vi "Main UI.vi"(11 "FormulaLV App in":refnum<class "FormulaG App.lvclass">) -> ()   [LabVIEW 2020, in "FormulaG.lvlib" / "FormulaG App.lvclass"]
uses:
  FormulaG App.lvclass
  <vilib>/sklein/WebView2/Webview2 Control/WebView2 Control.xctl
  FormulaLV-Common/Camera.ctl
  FormulaLV-Common/Car Info.ctl
  FormulaG App.lvclass/FormulaG App.ctl
  FormulaLV-Common/UI Options.ctl
  FormulaLV-Common/FormulaG-Common.lvlib
  FormulaG API/FormulaG API.lvclass
panel:
  out "XY Graph":cluster{dbl[], dbl[]}[](graph)
  out "Info":T1 {"Heading" format="%.2f"; "Y" format="%.2f"; "X" format="%.2f"; "Speed" format="%.2f"}
  in  "Pause":bool
  in  "Sensitivity":sgl(slide)=0.5148515 scale=0.0..1.0
  out "Chart":sgl[][](graph)
  in  "Camera":T2
  in  "Reset":bool
  in  "Throttle":sgl(slide)=0.16831683 scale=0.0..1.0
  out "Steering":sgl(knob) scale=-1.0..1.0
  out "Ranges":sgl[][](array[numeric]) format="%.2f"
  out "Connected":bool
  in  "Show Range Lines":bool
  out "Web":string(xcontrol)
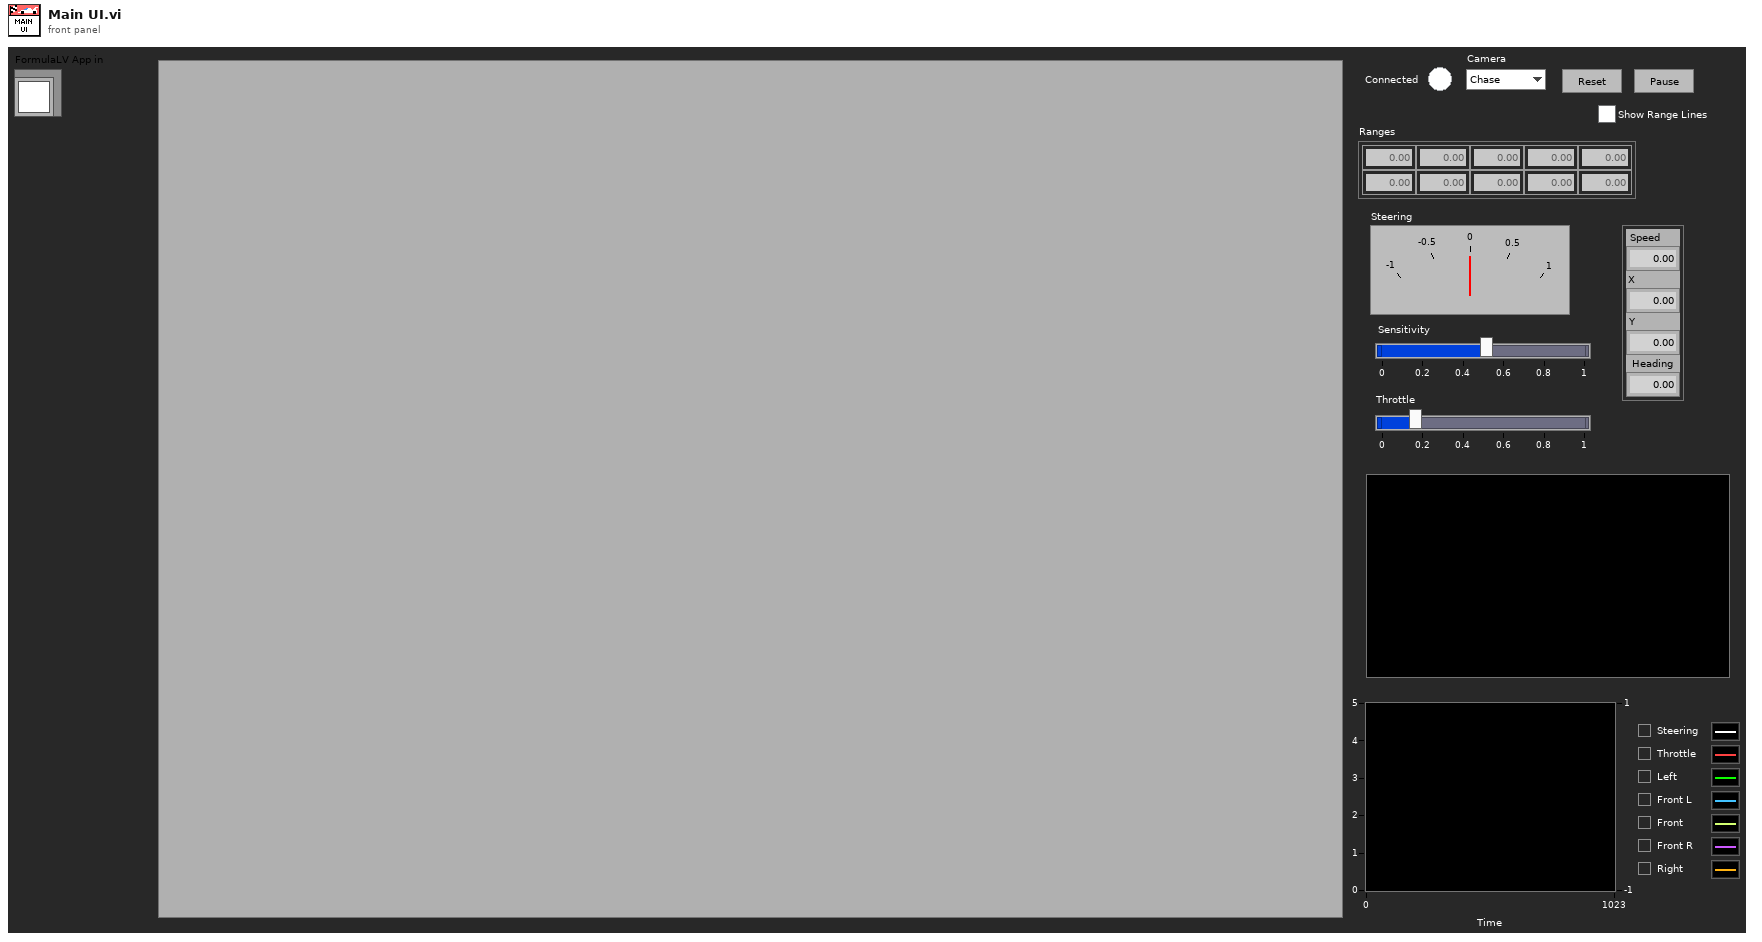
[diagram p1: front panel]
types:
  T1 = typedef "FormulaG-Common.lvlib/Car Info.ctl" = cluster{"Speed":sgl, "X":sgl, "Y":sgl, "Heading":sgl}
  T2 = typedef "FormulaG-Common.lvlib/Camera.ctl" = enum16{"Chase", "Overhead"}
  T3 = typedef "FormulaG-Common.lvlib/UI Options.ctl" = cluster{"Range Visible":bool}
  T4 = typedef "FormulaG-Common.lvlib/Ranges.ctl" = cluster{"Front":sgl[], "Rear":sgl[]}
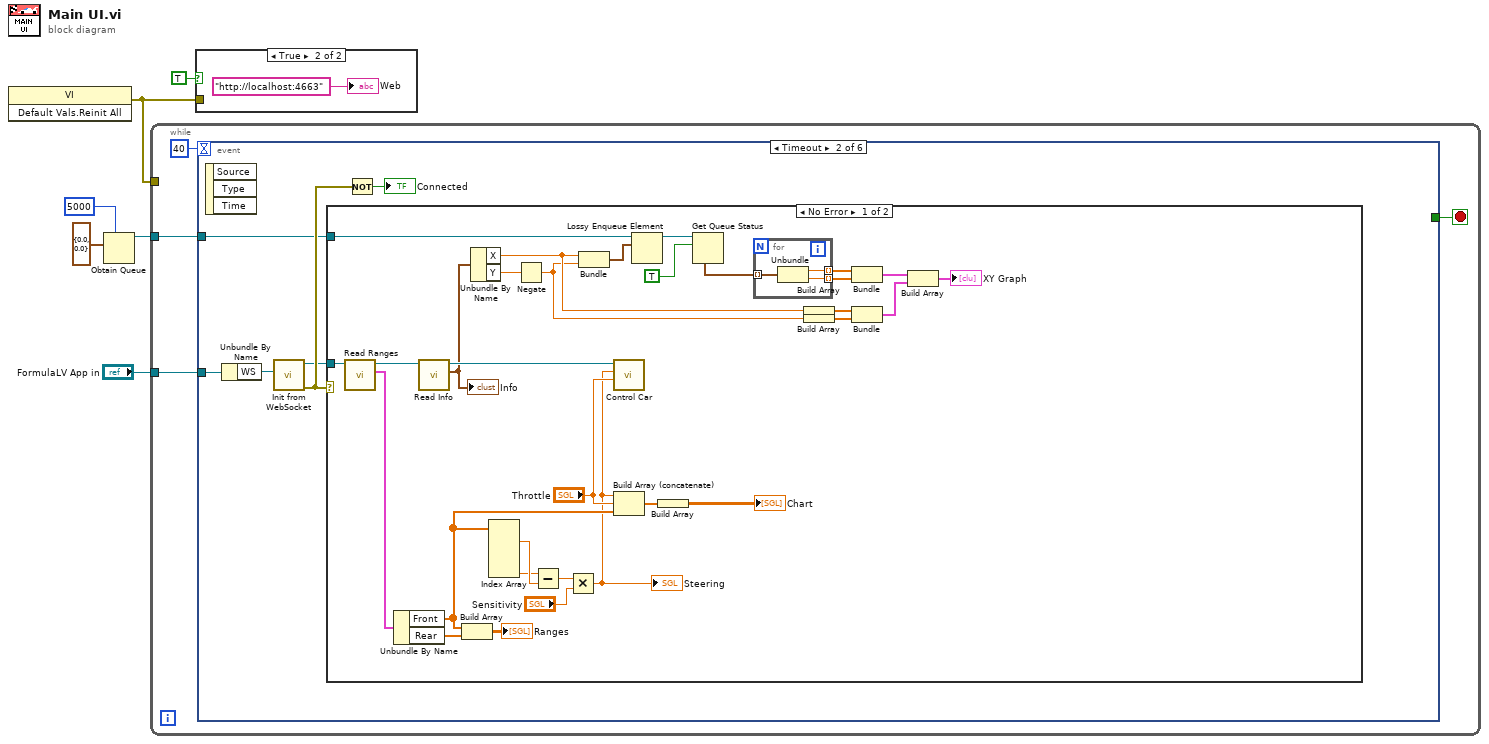
[diagram p0: block diagram]
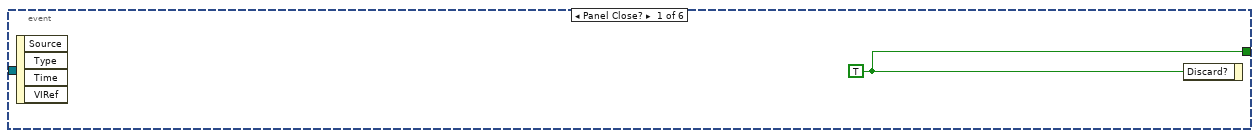
[diagram p3: hidden frame]
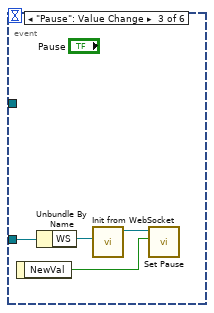
[diagram p5: hidden frame]
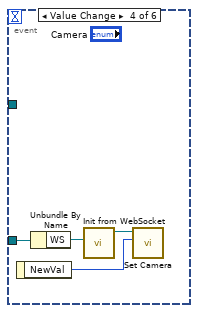
[diagram p6: hidden frame]
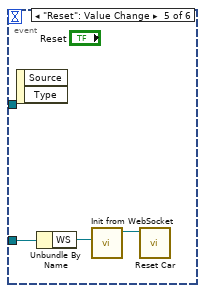
[diagram p7: hidden frame]
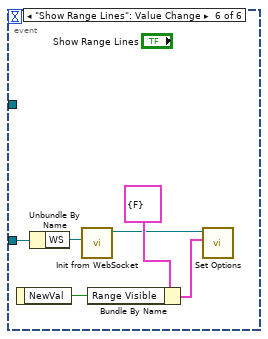
[diagram p8: hidden frame]
diagram:
  n1 = invoke class="VI" method="Default Vals.Reinit All"() -> (error out=w4:errorcluster)  [unwired: 3 in, 2 out]
  n2 = Obtain Queue(max queue size (-1, unlimited)=5000, element data type=cluster{dbl, dbl} {0.0, 0.0}) -> (queue out=w2:refnum<queue>)  [unwired: 3 in, 2 out]
  n3 = while {
    tunnel: "FormulaLV App in" -> [w9]
    tunnel: w4 -> [_]
    tunnel: w2 -> [w7]
    stop <- w10 stop-if-true
    n4 = event shown="[1] Timeout" {
      selector: _ -> [_ _ _ _ _ _]
      dyn-events: _ -> [_ _ _ _ _ _]
      timeout: 40 -> [_ _ _ _ _ _]
      tunnel: [w11 _ _ _ _ _] -> w10
      tunnel: w9 -> [_ w17 w55 w59 w62 w68]
      tunnel: w7 -> [_ w12 _ _ _ _]
      event Panel Close? {
        w11 = TRUE ("Discard?")
        n5 = event-data() -> ()  [unwired: 1 in, 4 out]
        n6 = event-data("Discard?"=w11) -> ()  [unwired: 1 in, 1 out]
      }
      event Timeout {
        n7 = event-data() -> ()  [unwired: 1 in, 3 out]
        n8 = Unbundle By Name(w17) -> ("WS"=w16:refnum<class "Websocket Server.lvclass">)
        n9 = call "Init from WebSocket.vi"("WS"=w16) -> ("error out"=w14:errorcluster, "FormulaG API out"=w13:refnum<class "FormulaG API.lvclass">)  [unwired: 9 in]
        n10 = case shown="No Error" w14 {
          tunnel: w13 -> [w44 _]
          tunnel: w12 -> [w31 _]
          frame No Error {
            n11 = call "Read Ranges.vi"("FormulaG API in"=w44) -> ("Ranges"=w43:T4, "FormulaG API out"=w39:refnum<class "FormulaG API.lvclass">)  [unwired: 8 in, 1 out]
            n12 = Unbundle By Name(w43) -> ("Front"=w41:sgl[], "Rear"=w42:sgl[])
            n13 = call "Read Info.vi"("FormulaG API in"=w39) -> ("Info"=w33:T1, "FormulaG API out"=w34:refnum<class "FormulaG API.lvclass">)  [unwired: 8 in, 1 out]
            "Info" <- w33
            n14 = Build Array(w41, w42) -> (→"Ranges":sgl[][])
            n15 = Unbundle By Name(w33) -> ("X"=w27:sgl, "Y"=w32:sgl)
            n16 = Index Array(array=w41) -> (element #1=w46:sgl, element #5=w45:sgl)  [unwired: 5 in, 3 out]
            n17 = Negate(x=w32) -> (-x=w26:sgl)
            n18 = Subtract(x=w45, y=w46) -> (x-y=w47:sgl)
            n19 = Multiply(x=w47, y="Sensitivity") -> (x*y=w37:sgl)
            "Steering" <- w37
            n20 = Bundle("X"=w27, w26) -> (w30:cluster{"X":sgl, sgl})  [unwired: 1 in]
            n21 = call "Control Car.vi"("Throttle"="Throttle", "Steering"=w37, "FormulaG API in"=w34) -> ()  [unwired: 7 in, 2 out]
            n22 = Build Array (concatenate)(w37, "Throttle", w41) -> (w36:sgl[])
            n23 = Lossy Enqueue Element(queue=w31, element=w30) -> (queue out=w29:refnum<queue>)  [unwired: 1 in, 3 out]
            n24 = Build Array(w36) -> (→"Chart":sgl[][])
            n25 = Get Queue Status(queue=w29, return elements? (F)=TRUE) -> (elements=w25:cluster{dbl, dbl}[])  [unwired: 1 in, 7 out]
            n26 = for {
              tunnel: w25 -> [w51] mode=indexing
              tunnel: [w50] -> w22 mode=indexing
              tunnel: [w49] -> w21 mode=indexing
              n27 = Unbundle(w51) -> (w50:dbl, w49:dbl)
            }
            n28 = Build Array(w27) -> (w24:sgl[])
            n29 = Build Array(w26) -> (w23:sgl[])
            n30 = Bundle(w22, w21) -> (w20:cluster{dbl[], dbl[]})  [unwired: 1 in]
            n31 = Bundle(w24, w23) -> (w19:cluster{sgl[], sgl[]})  [unwired: 1 in]
            n32 = Build Array(w20, w19) -> (→"XY Graph":cluster{dbl[], dbl[]}[])
          }
          frame Error {
          }
        }
        n33 = Not(x=w14) -> (.not. x?=→"Connected":bool)
      }
      event "Pause": Value Change {
        n34 = event-data() -> ("NewVal"=w52:bool)  [unwired: 1 in]
        n35 = Unbundle By Name(w55) -> ("WS"=w54:refnum<class "Websocket Server.lvclass">)
        n36 = call "Init from WebSocket.vi"("WS"=w54) -> ("FormulaG API out"=w53:refnum<class "FormulaG API.lvclass">)  [unwired: 9 in, 1 out]
        n37 = call "Set Pause.vi"("Pause"=w52, "FormulaG API in"=w53) -> ()  [unwired: 8 in, 2 out]
      }
      event Value Change {
        n38 = event-data() -> ("NewVal"=w56:T2)  [unwired: 1 in]
        n39 = Unbundle By Name(w59) -> ("WS"=w58:refnum<class "Websocket Server.lvclass">)
        n40 = call "Init from WebSocket.vi"("WS"=w58) -> ("FormulaG API out"=w57:refnum<class "FormulaG API.lvclass">)  [unwired: 9 in, 1 out]
        n41 = call "Set Camera.vi"("Camera"=w56, "FormulaG API in"=w57) -> ()  [unwired: 8 in, 2 out]
      }
      event "Reset": Value Change {
        n42 = event-data() -> ()  [unwired: 1 in, 2 out]
        n43 = Unbundle By Name(w62) -> ("WS"=w61:refnum<class "Websocket Server.lvclass">)
        n44 = call "Init from WebSocket.vi"("WS"=w61) -> ("FormulaG API out"=w60:refnum<class "FormulaG API.lvclass">)  [unwired: 9 in, 1 out]
        n45 = call "Reset Car.vi"("FormulaG API in"=w60) -> ()  [unwired: 9 in, 2 out]
      }
      event "Show Range Lines": Value Change {
        n46 = event-data() -> ("NewVal"=w66:bool)  [unwired: 1 in]
        n47 = Unbundle By Name(w68) -> ("WS"=w65:refnum<class "Websocket Server.lvclass">)
        n48 = call "Init from WebSocket.vi"("WS"=w65) -> ("FormulaG API out"=w64:refnum<class "FormulaG API.lvclass">)  [unwired: 9 in, 1 out]
        n49 = Bundle By Name(cluster=T3 {"Range Visible"=FALSE} ("UI Options"), "Range Visible"=w66) -> (w63:T3)
        n50 = call "Set Options.vi"("UI Options"=w63, "FormulaG API in"=w64) -> ()  [unwired: 8 in, 2 out]
      }
    }
  }
  n51 = case shown="True" TRUE {
    tunnel: w4 -> [_ _]
    frame False {
    }
    frame True {
      "Web" <- "http://localhost:4663" ("Web")
    }
  }
